vi "JKI State Machine Helper - VI Tree.vi"   [LabVIEW 2013]
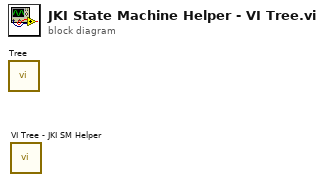
[diagram p0: block diagram]
diagram:
  n1 = call "Tree.vi"() -> ()  [unwired: 1 in]
  n2 = call "VI Tree - JKI SM Helper.vi"() -> ()  [unwired: 12 in]
